vi "DisplayOneFrame.vi"(7 "handle":u64, 8 "error in (no error)":errorcluster caption="错误输入（无错误）", 9 "pstDisplayInfo In":T1, 10 "pData In":u8[](array[numeric]), 11 "hWnd":u64[](array[numeric])) -> (0 "error out":errorcluster caption="错误输出", 1 "pstDisplayInfo Out":T1, 3 "function return":i32, 5 "handle out":u64)   [LabVIEW 2015, in "MvCameraControl.lvlib"]
doc: "MV_LV_API int __stdcall SaveImage(MV_SAVE_IMAGE_PARAM* pSaveParam);"
uses:
  MvCameraControl.lvlib
  MvCameraPatch.dll
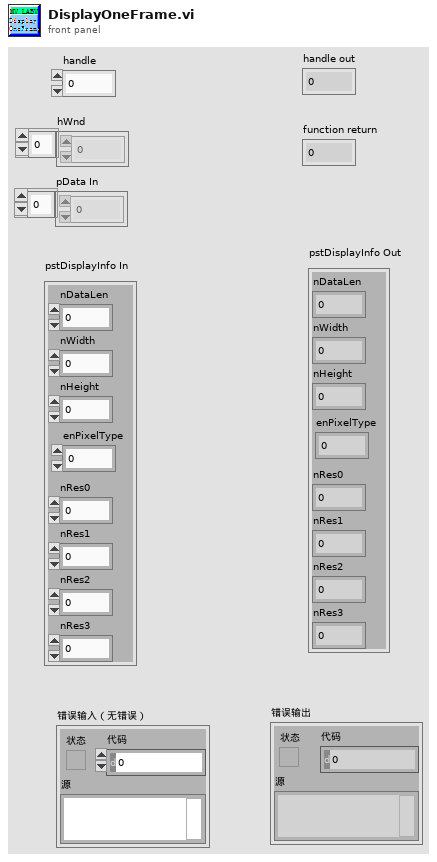
[diagram p1: front panel]
types:
  T1 = cluster{"nDataLen":u16, "nWidth":u16, "nHeight":u32, "enPixelType":u32, "nRes0":u32, "nRes1":u32, "nRes2":u32, "nRes3":u32}
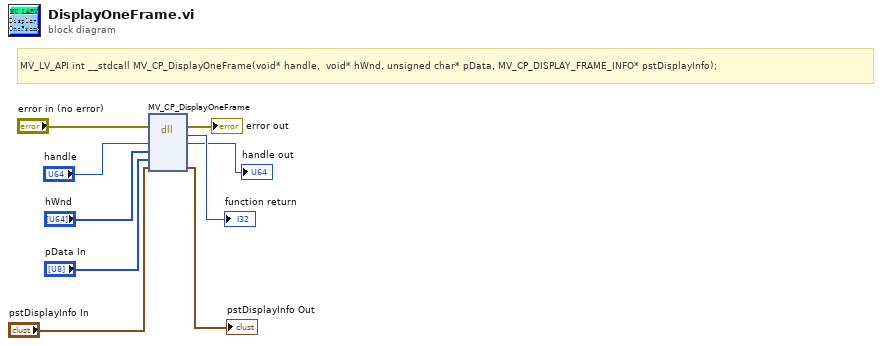
[diagram p0: block diagram]
diagram:
  # "MV_LV_API int __stdcall MV_CP_DisplayOneFrame(void* handle,  void* hWnd, unsigned char* pData, MV_CP_DISPLAY_FRAME_INFO* pstDisplayInfo);"
  n1 = dll-call lib="MvCameraPatch.dll" fn="MV_CP_DisplayOneFrame"(error in="error in (no error)", "handle"="handle", "hWnd"="hWnd", "pData"="pData In", "pstDisplayInfo"="pstDisplayInfo In") -> (error out=→"error out":errorcluster, "返回类型"=→"function return":i32, "handle"=→"handle out":u64, "pstDisplayInfo"=→"pstDisplayInfo Out":T1)  [unwired: 4 in, 1 out]
